vi "Kompatator 3.0..vi"() -> ()   [LabVIEW 2020]
panel:
  out "P>Q?":bool
  out "P=Q?":bool
  in  "Q":dbl
  in  "P":dbl
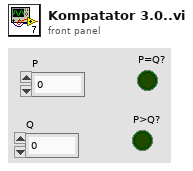
[diagram p1: front panel]
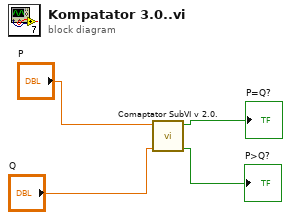
[diagram p0: block diagram]
diagram:
  n1 = call "Comaptator SubVI v 2.0..vi"("Q"="Q", "P"="P") -> ("P>Q?"=→"P>Q?":bool, "P=Q?"=→"P=Q?":bool)  [unwired: 8 in]
